vi "From Variant.vi"(8 "Error In":errorcluster, 10 "Variant":variant, 11 "TD Int In":refnum<class "Int.lvclass">) -> (0 "Error Out":errorcluster, 3 "TD Int Out":refnum<class "Int.lvclass">)   [LabVIEW 2020, in "NI_VIAnCFGDataStructure.lvlib" / "Int.lvclass"]
doc: "Dynamic dispatch interface for conversion of variant LV data to Tree Data classes."
uses:
  <vilib>/addons/analyzer/VIAnCFGDataStructure/Data Types/Int/Int.lvclass
  <vilib>/addons/analyzer/VIAnCFGDataStructure/Data Types/Int/Int.lvclass/Int.ctl
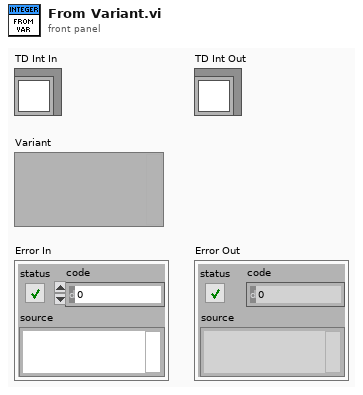
[diagram p1: front panel]
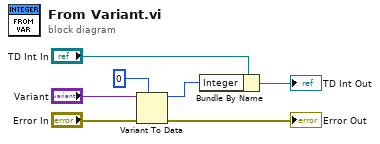
[diagram p0: block diagram]
diagram:
  n1 = Variant To Data(error in="Error In", type=i64 0 ("Integer"), Variant="Variant") -> (data=w2:i64, error out=→"Error Out":errorcluster)
  n2 = Bundle By Name(cluster="TD Int In", "Integer"=w2) -> (→"TD Int Out":refnum<class "Int.lvclass">)
